vi "Facade.vi"(0 "Data In":T5, 2 "Display State In":T3, 3 "Container State":T4) -> (6 "Data Out":T5, 7 "Display State Out":T3, 8 "Action":T2)   [LabVIEW 2020, in "Timeout XCtrl.xctl"]
uses:
  Timeout XCtrl.xctl
  <vilib>/_xctls/Action.ctl
  <vilib>/_xctls/XControlSupport.lvlib
  Classes/Timeout/Timeout.lvclass
  epl-vi-lib/Utility VIs/Error Handling VIs/Error-Library Action.ctl
  <vilib>/_xctls/Container State.ctl
  Data.vi
  State.vi
panel:
  in  "Color Box":u32(colorbox)
  in  "Result":string
  in  "Tabs":enum32{"Hist", "Msg"}(tab)
  out "histogram":T1(graph)
  out "X-axis":dbl(slide) scale=0.0..4.75
  out "Message":string
  in  "Expr":string caption="State times out after"
  in  "Units":enum16{"reps", "sec"}(ring)
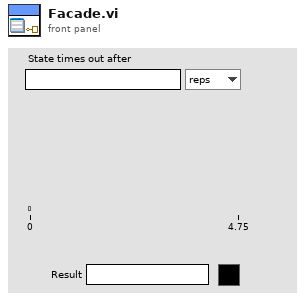
[diagram p1: front panel]
types:
  T1 = cluster{"X Values":dbl[], "Histogram: h(x)":dbl[]}[]
  T2 = typedef "XControlSupport.lvlib/Action.ctl" = cluster{"Data Changed?":bool, "State Changed?":bool, "Action Name":string}
  T3 = typedef "Timeout XCtrl.xctl/State.vi" = cluster{"plot":bool}
  T4 = typedef "XControlSupport.lvlib/Container State.ctl" = cluster{"Indicator?":bool, "Run Mode?":bool, " Refnum":refnum<vi>}
  T5 = typedef "Timeout XCtrl.xctl/Data.vi" = refnum<class "Timeout.lvclass">
  T6 = typedef "Error-Library Action.ctl" = enum16{"NONE", "Register", "Read"}
  T7 = typedef "Error Description.ctl" = cluster{"Code":i32, "Description":string, "Details":string}
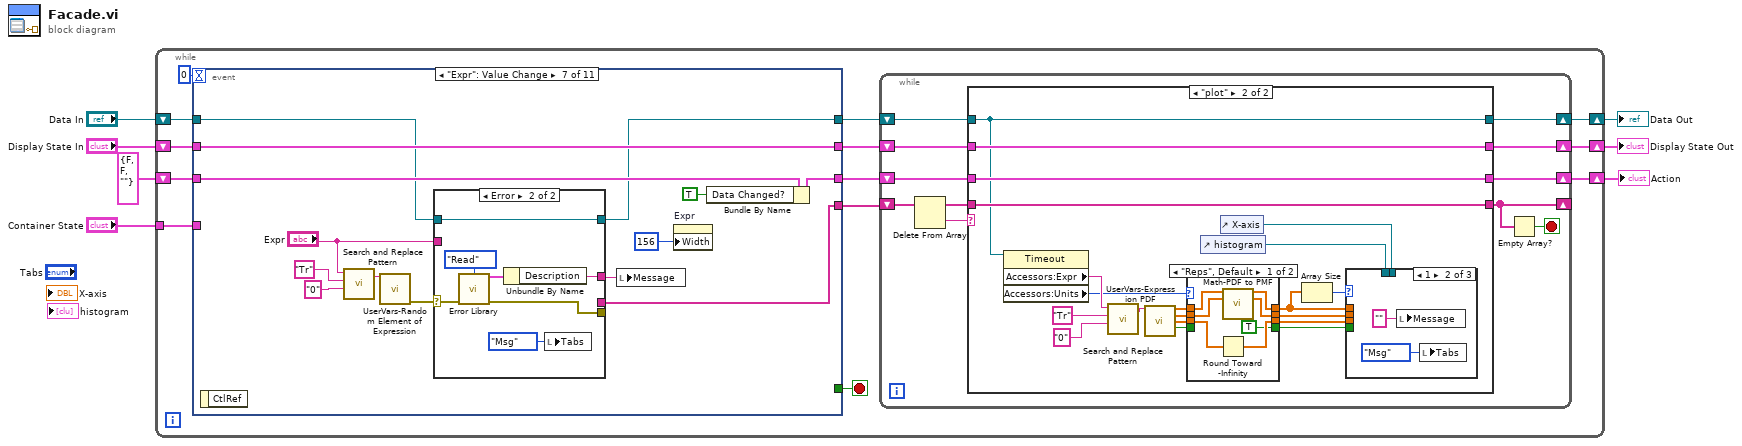
[diagram p0: block diagram]
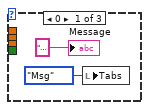
[diagram p4: hidden frame]
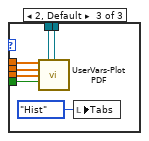
[diagram p5: hidden frame]
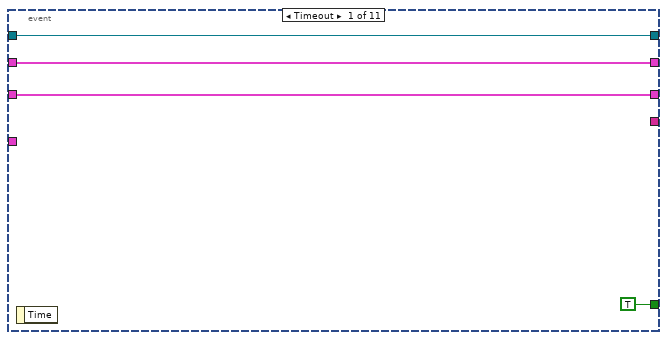
[diagram p6: hidden frame]
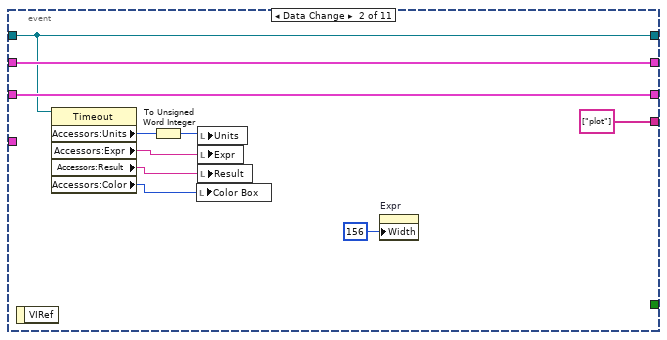
[diagram p7: hidden frame]
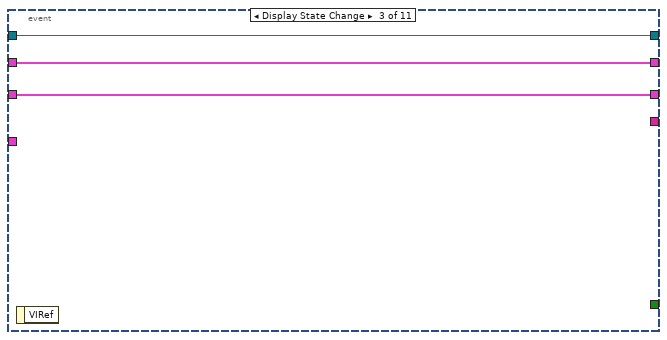
[diagram p8: hidden frame]
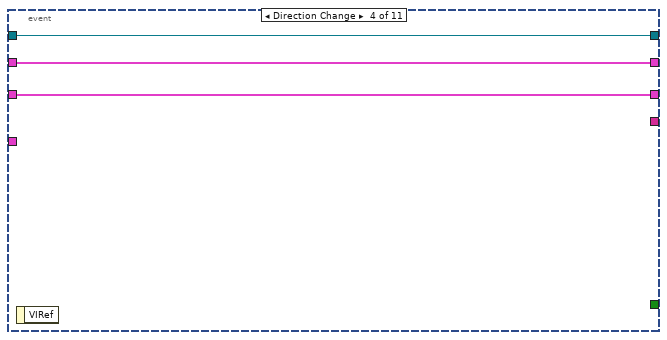
[diagram p9: hidden frame]
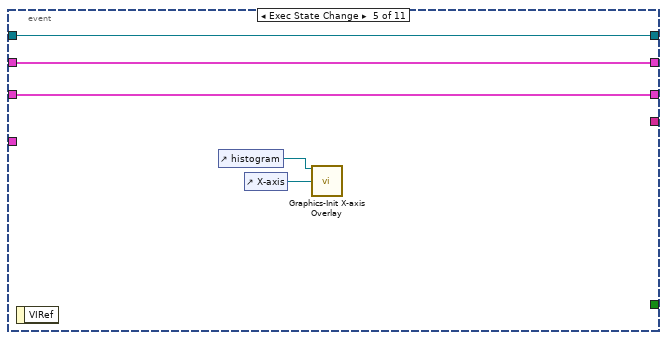
[diagram p10: hidden frame]
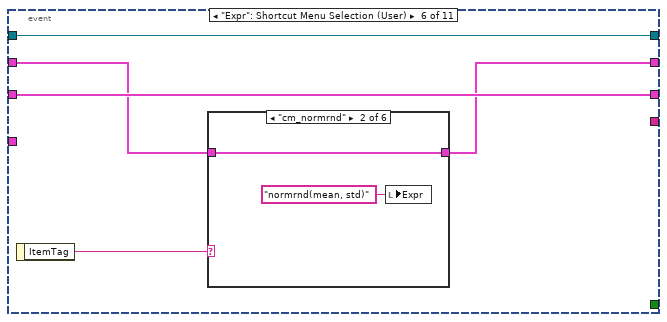
[diagram p11: hidden frame]
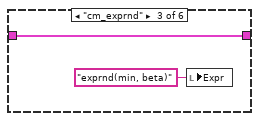
[diagram p13: hidden frame]
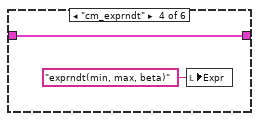
[diagram p14: hidden frame]
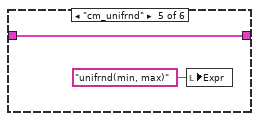
[diagram p15: hidden frame]
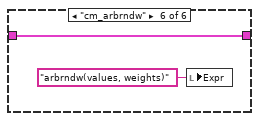
[diagram p16: hidden frame]
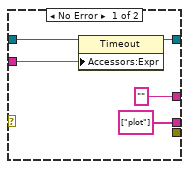
[diagram p17: hidden frame]
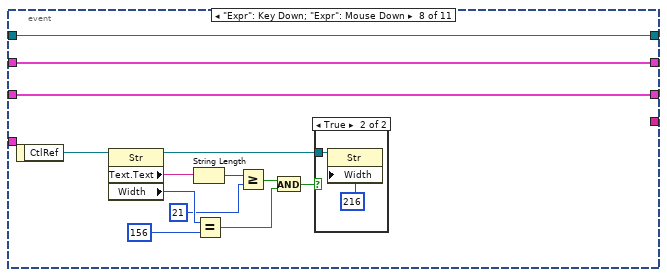
[diagram p18: hidden frame]
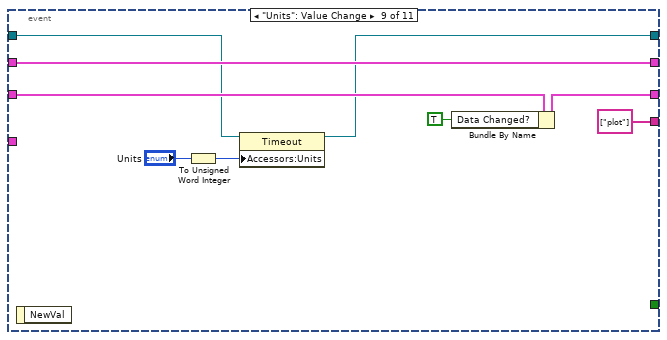
[diagram p20: hidden frame]
diagram:
  n1 = while {
    shift-right: [w10] -> w4
    shift-left: "Display State In" -> [w20]
    tunnel: "Container State" -> [w17]
    shift-right: [w11] -> w7
    shift-left: "Data In" -> [w16]
    shift-right: [w9] -> w2
    shift-left: T2 {"Data Changed?"=FALSE, "State Changed?"=FALSE, "Action Name"=""} ("Action") -> [w15]
    stop <- w19 stop-if-true
    n2 = event shown="[6] \"Expr\": Value Change" {
      selector: _ -> [_ _ _ _ _ _ _ _ _ _ _]
      dyn-events: _ -> [_ _ _ _ _ _ _ _ _ _ _]
      timeout: 0 -> [_ _ _ _ _ _ _ _ _ _ _]
      tunnel: w20 -> [w79 w91 w94 w97 w102 w104 w132 w157 w168 w175 w182]
      tunnel: [w79 w91 w94 w97 w102 w103 w132 w157 w168 w175 w182] -> w13
      tunnel: [TRUE _ _ _ _ _ _ _ _ _ _] -> w19
      tunnel: w17 -> [_ _ _ _ _ _ _ _ _ _ _]
      tunnel: w16 -> [w78 w88 w93 w96 w101 w107 w123 w156 w165 w173 w180]
      tunnel: [w78 w88 w93 w96 w101 w107 w122 w156 w164 w172 w179] -> w12
      tunnel: [w80 w90 w92 w95 w100 w106 w120 w155 w161 w171 w178] -> w14
      tunnel: w15 -> [w80 w90 w92 w95 w100 w106 w131 w155 w167 w174 w181]
      tunnel: [_ string[] ["plot"] _ _ _ _ w121 _ string[] ["plot"] _ _] -> w8
      event Timeout {
        n3 = event-data() -> ()  [unwired: 1 in, 1 out]
      }
      event Data Change {
        n4 = event-data() -> ()  [unwired: 1 in, 1 out]
        n5 = property class="Timeout"(reference=w88) -> ("Accessors:Units"=w87:enum16{"Reps", "Seconds"}, "Accessors:Expr"=w85:string, "Accessors:Result"=w83:string, "Accessors:Color"=w82:u32)  [unwired: 1 in, 2 out]
        n6 = To Unsigned Word Integer(number=w87) -> (unsigned 16bit integer=w86:u16)
        n7 = local write "Color Box"(w82) -> ()
        n8 = local write "Units"(w86) -> ()
        n9 = local write "Expr"(w85) -> ()
        n10 = local write "Result"(w83) -> ()
        n11 = property on="Expr" class="Str"("Width"=u32 156 ("Size:Width")) -> ()  [unwired: 2 in, 2 out]
      }
      event Display State Change {
        n12 = event-data() -> ()  [unwired: 1 in, 1 out]
      }
      event Direction Change {
        n13 = event-data() -> ()  [unwired: 1 in, 1 out]
      }
      event Exec State Change {
        n14 = event-data() -> ()  [unwired: 1 in, 1 out]
        n15 = control-ref of="histogram"() -> (w98:refnum<vi>)
        n16 = control-ref of="X-axis"() -> (w99:refnum<vi>)
        n17 = call "Graphics-Init X-axis Overlay.vi"("Ctl Refnum"=w98, "X-axis slider"=w99) -> ()  [unwired: 13 in, 1 out]
      }
      event "Expr": Shortcut Menu Selection (User) {
        n18 = event-data() -> ("ItemTag"=w105:string)  [unwired: 1 in]
        n19 = case shown="\"cm_normrnd\"" w105 {
          tunnel: w104 -> [w108 w109 w111 w113 w115 w117]
          tunnel: [w108 w109 w111 w113 w115 w117] -> w103
          frame "False", Default {
          }
          frame "cm_normrnd" {
            n20 = local write "Expr"("normrnd(mean, std)" ("Expr")) -> ()
          }
          frame "cm_exprnd" {
            n21 = local write "Expr"("exprnd(min, beta)" ("Expr")) -> ()
          }
          frame "cm_exprndt" {
            n22 = local write "Expr"("exprndt(min, max, beta)" ("Expr")) -> ()
          }
          frame "cm_unifrnd" {
            n23 = local write "Expr"("unifrnd(min, max)" ("Expr")) -> ()
          }
          frame "cm_arbrndw" {
            n24 = local write "Expr"("arbrndw(values, weights)" ("Expr")) -> ()
          }
        }
      }
      event "Expr": Value Change {
        n25 = event-data() -> ()  [unwired: 1 in, 1 out]
        n26 = call <vilib>:"Search and Replace Pattern.vi"("string"="Expr", "regular expression (\"\")"="Tr" ("regular expression (\"\")"), "replace string (\"\")"="0" ("replace string (\"\")")) -> ("result string"=w126:string)  [unwired: 2 in, 1 out]
        n27 = call "UserVars-Random Element of Expression.vi"("Expr"=w126) -> ("error out"=w130:errorcluster)  [unwired: 12 in, 2 out]
        n28 = case shown="Error" w130 {
          selector: w130 -> [_ w144]
          tunnel: "Expr" -> [w135 _]
          tunnel: ["" ("Description") w138] -> w129
          tunnel: [_ w142] -> _
          tunnel: w123 -> [w136 w141]
          tunnel: [w134 w141] -> w122
          tunnel: [string[] ["plot"] _] -> w121
          frame No Error {
            n29 = property class="Timeout"(reference=w136, "Accessors:Expr"=w135) -> (reference out=w134:T5)  [unwired: 1 in, 1 out]
          }
          frame Error {
            n30 = call "Error Library.vi"("action"=Error-Library_Action."Read", "error in"=w144) -> ("Entry"=w143:T7, "error thru"=w142:errorcluster)  [unwired: 11 in, 1 out]
            n31 = Unbundle By Name(w143) -> ("Description"=w138:string)
            n32 = local write "Tabs"(enum32{"Hist", "Msg"}."Msg" ("Tabs")) -> ()
          }
        }
        n33 = local write "Message"(w129) -> ()
        n34 = property on="Expr" class="Str"("Width"=u32 156 ("Size:Width")) -> ()  [unwired: 2 in, 2 out]
        n35 = Bundle By Name(cluster=w131, "Data Changed?"=TRUE) -> (w120:T2)
      }
      event "Expr": Key Down; "Expr": Mouse Down {
        n36 = event-data() -> ("CtlRef"=w146:refnum<vi>)  [unwired: 1 in]
        n37 = property class="Str"(reference=w146) -> (reference out=w154:refnum<vi>, "Text.Text"=w147:string, "Width"=w151:u32)  [unwired: 1 in, 1 out]
        n38 = String Length(string=w147) -> (length=w148:i32)
        n39 = Equal?(x=w151, y=u32 156) -> (x = y?=w153:bool)
        n40 = Greater Or Equal?(x=w148, y=21) -> (x >= y?=w150:bool)
        n41 = And(x=w150, y=w153) -> (x .and. y?=w145:bool)
        n42 = case shown="True" w145 {
          tunnel: w154 -> [_ w159]
          frame False {
          }
          frame True {
            n43 = property class="Str"(reference=w159, "Width"=u32 216 ("y")) -> ()  [unwired: 1 in, 2 out]
          }
        }
      }
      event "Units": Value Change {
        n44 = event-data() -> ()  [unwired: 1 in, 1 out]
        n45 = To Unsigned Word Integer(number="Units") -> (unsigned 16bit integer=w163:u16)
        n46 = property class="Timeout"(reference=w165, "Accessors:Units"=w163) -> (reference out=w164:T5)  [unwired: 1 in, 1 out]
        n47 = Bundle By Name(cluster=w167, "Data Changed?"=TRUE) -> (w161:T2)
      }
      event "Result": Value Change {
        n48 = event-data() -> ()  [unwired: 1 in, 1 out]
        n49 = property class="Timeout"(reference=w173, "Accessors:Result"="Result") -> (reference out=w172:T5)  [unwired: 1 in, 1 out]
        n50 = Bundle By Name(cluster=w174, "Data Changed?"=TRUE) -> (w171:T2)
      }
      event "Color Box": Value Change {
        n51 = event-data() -> ()  [unwired: 1 in, 1 out]
        n52 = property class="Timeout"(reference=w180, "Accessors:Color"="Color Box") -> (reference out=w179:T5)  [unwired: 1 in, 1 out]
        n53 = Bundle By Name(cluster=w181, "Data Changed?"=TRUE) -> (w178:T2)
      }
    }
    n54 = while {
      shift-right: [w28] -> _
      shift-left: w8 -> [w31]
      shift-right: [w26] -> w11
      shift-left: w12 -> [w25]
      shift-right: [w24] -> w10
      shift-left: w13 -> [w23]
      shift-right: [w21] -> w9
      shift-left: w14 -> [w22]
      stop <- w27 stop-if-true
      n55 = Delete From Array(array=w31) -> (deleted portion=w29:string, array with subset deleted=w30:string[])  [unwired: 2 in]
      n56 = case shown="\"plot\"" w29 {
        tunnel: w30 -> [w35 w55]
        tunnel: [w35 w55] -> w28
        tunnel: [w32 w40] -> w26
        tunnel: w25 -> [w32 w40]
        tunnel: [w33 w54] -> w24
        tunnel: w23 -> [w33 w54]
        tunnel: w22 -> [w34 w53]
        tunnel: [w34 w53] -> w21
        frame "", Default {
        }
        frame "plot" {
          n57 = property class="Timeout"(reference=w40) -> ("Accessors:Expr"=w39:string, "Accessors:Units"=w38:enum16{"Reps", "Seconds"})  [unwired: 1 in, 2 out]
          n58 = call <vilib>:"Search and Replace Pattern.vi"("string"=w39, "regular expression (\"\")"="Tr" ("regular expression (\"\")"), "replace string (\"\")"="0" ("replace string (\"\")")) -> ("result string"=w41:string)  [unwired: 2 in, 1 out]
          n59 = call "UserVars-Expression PDF.vi"("Expr"=w41) -> ("X"=w52:dbl[], "PDF"=w51:dbl[], "refpts"=w50:dbl[], "mass function"=w49:bool)  [unwired: 10 in, 1 out]
          n60 = case shown="\"Reps\", Default" w38 {
            tunnel: w52 -> [w59 w66]
            tunnel: w51 -> [w57 w65]
            tunnel: w50 -> [w62 w64]
            tunnel: [w58 w66] -> w37
            tunnel: [w56 w65] -> w46
            tunnel: [w61 w64] -> w45
            tunnel: w49 -> [_ w63]
            tunnel: [TRUE ("mass function") w63] -> w44
            frame "Reps", Default {
              n61 = Round Toward -Infinity(1:w62) -> (0:w61:dbl[])
              n62 = call "Math-PDF to PMF.vi"("X in"=w59, "PDF"=w57) -> ("X out"=w58:dbl[], "PMF"=w56:dbl[])  [unwired: 12 in]
            }
            frame "Seconds" {
            }
          }
          n63 = control-ref of="histogram"() -> (w47:refnum<vi>)
          n64 = control-ref of="X-axis"() -> (w48:refnum<vi>)
          n65 = Array Size(array=w37) -> (size(s)=w36:i32)
          n66 = case shown="1" w36 {
            tunnel: w48 -> [_ _ w77]
            tunnel: w47 -> [_ _ w76]
            tunnel: w37 -> [_ _ w72]
            tunnel: w46 -> [_ _ w75]
            tunnel: w45 -> [_ _ w74]
            tunnel: w44 -> [_ _ w73]
            frame 0 {
              n67 = local write "Tabs"(enum32{"Hist", "Msg"}."Msg" ("Tabs")) -> ()
              "Message" <- "Distribution too complicated to display." ("Value (Signaling)")
            }
            frame 1 {
              n68 = local write "Message"("") -> ()
              n69 = local write "Tabs"(enum32{"Hist", "Msg"}."Msg" ("Tabs")) -> ()
            }
            frame 2, Default {
              n70 = call "UserVars-Plot PDF.vi"("X"=w72, "XYGraph"=w76, "X-axis"=w77, "PDF"=w75, "refpts"=w74, "mass"=w73) -> ()  [unwired: 10 in]
              n71 = local write "Tabs"(enum32{"Hist", "Msg"}."Hist" ("Tabs")) -> ()
            }
          }
        }
      }
      n72 = Empty Array?(array=w28) -> (empty?=w27:bool)
    }
  }
  "Display State Out" <- w4
  "Data Out" <- w7
  "Action" <- w2
